vi "Draw Wiggle Trace.vi"(5 "Offsets":cluster{"X offset":u32, "Y offset":u32}, 6 "Trace Options":T1={"Trace Amplitude"=1.0, "Trace Color"=16448250, "Fill options"=enum."No Fill"}, 7 "Plot Area Size":cluster{"Width":u32, "Height":u32}, 8 "error in (no error)":errorcluster, 10 "Data":dbl[][](array[numeric]), 11 "picture in":picture) -> (0 "error out":errorcluster, 3 "picture out":picture)   [LabVIEW 2009]
uses:
  Controls/Trace Options.ctl
  Controls/Fill Options.ctl
  <vilib>/Analysis/baseanly.llb/Quick Scale 2D.vi
  <vilib>/Analysis/NI_AALBase.lvlib
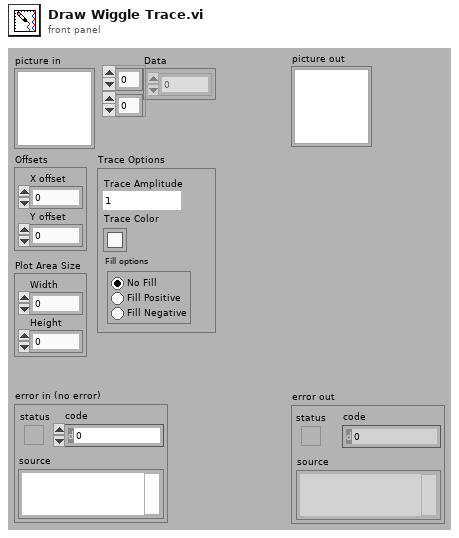
[diagram p1: front panel]
types:
  T1 = typedef "Trace Options.ctl" = cluster{"Trace Amplitude":dbl, "Trace Color":u32, "Fill options":T2}
  T2 = typedef "Fill Options.ctl" = enum32{"No Fill", "Fill Positive", "Fill Negative"}
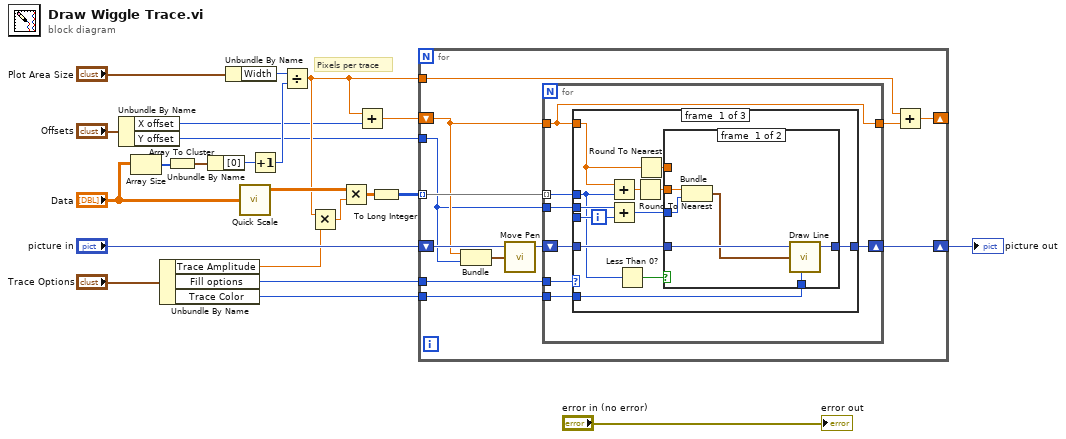
[diagram p0: block diagram]
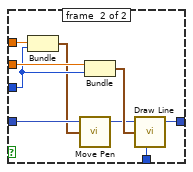
[diagram p2: hidden frame]
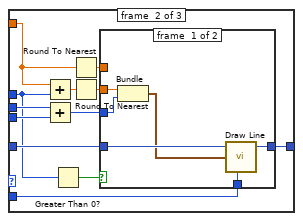
[diagram p3: hidden frame]
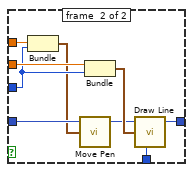
[diagram p4: hidden frame]
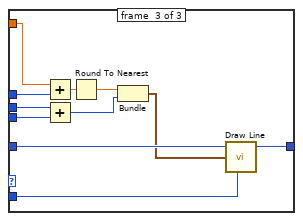
[diagram p5: hidden frame]
diagram:
  # "Pixels per trace"
  n1 = Unbundle By Name("Offsets") -> ("X offset"=w11:u32, "Y offset"=w10:u32)
  n2 = Array Size(array="Data") -> (size(s)=w8:i32[])
  n3 = Unbundle By Name("Trace Options") -> ("Trace Amplitude"=w4:dbl, "Fill options"=w2:T2, "Trace Color"=w1:u32)
  n4 = Array To Cluster(array=w8) -> (cluster=w6:cluster{"[0]":i32, "[1]":i32})
  n5 = Unbundle By Name(w6) -> ("[0]"=w19:i32)
  n6 = Unbundle By Name("Plot Area Size") -> ("Width"=w12:u32)
  n7 = call-poly <vilib>:"Quick Scale.vi"("X"="Data") -> ("Yij=Xij/Max|X|"=w23:dbl[][])  [unwired: 2 out]
  n8 = Increment(x=w19) -> (x+1=w17:i32)
  n9 = Divide(x=w12, y=w17) -> (x/y=w21:dbl)
  n10 = Multiply(x=w21, y=w4) -> (x*y=w22:dbl)
  n11 = Multiply ("Multiply.vi")(x=w23, y=w22) -> (x*y=w15:dbl[][])
  n12 = Add(x=w21, y=w11) -> (x+y=w18:dbl)
  n13 = To Long Integer(number=w15) -> (32bit integer=w14:i32[][])
  n14 = for {
    tunnel: w14 -> [w35] mode=indexing
    tunnel: w21 -> [w32]
    shift-right: [w31] -> _
    shift-left: w18 -> [w28]
    shift-right: [w34] -> w13
    shift-left: "picture in" -> [w30]
    tunnel: w10 -> [w26]
    tunnel: w2 -> [w25]
    tunnel: w1 -> [w24]
    n15 = Bundle(w28, "Y offset"=w26) -> (w27:cluster{dbl, "Y offset":u32})  [unwired: 1 in]
    n16 = call <vilib>:"Move Pen.vi"("new position"=w27, "picture"=w30) -> ("new picture"=w29:picture)  [unwired: 3 in]
    n17 = for {
      tunnel: w35 -> [w39] mode=indexing
      tunnel: w28 -> [w38]
      shift-right: [w43] -> w34
      shift-left: w29 -> [w42]
      tunnel: [w38] -> w33
      tunnel: w26 -> [w40]
      tunnel: w25 -> [w36]
      tunnel: w24 -> [w37]
      i -> [w41]
      n18 = case shown="\"Fill Negative\"" w36 {
        tunnel: [w55 w82 w108] -> w43
        tunnel: w42 -> [w54 w81 w107]
        tunnel: w41 -> [w53 w80 w106]
        tunnel: w40 -> [w51 w78 w104]
        tunnel: w39 -> [w49 w76 w102]
        tunnel: w38 -> [w47 w74 w100]
        tunnel: w37 -> [w45 w72 w99]
        frame #0 {
          n19 = Add(x=w47, y=w49) -> (x+y=w48:dbl)
          n20 = Add(x=w51, y=w53) -> (x+y=w52:u32)
          n21 = Less Than 0?(x=w49) -> (x < 0?=w44:bool)
          n22 = Round To Nearest(number=w48) -> (nearest integer value=w50:dbl)
          n23 = Round To Nearest(number=w47) -> (nearest integer value=w46:dbl)
          n24 = case shown="True" w44 {
            tunnel: [w61 w70] -> w55
            tunnel: w54 -> [w60 w67]
            tunnel: w52 -> [w58 w64]
            tunnel: w50 -> [w57 w68]
            tunnel: w46 -> [_ w65]
            tunnel: w45 -> [w56 w62]
            frame #0 {
              n25 = Bundle(w57, w58) -> (w59:cluster{dbl, u32})  [unwired: 1 in]
              n26 = call <vilib>:"Draw Line.vi"("picture"=w60, "end point"=w59, "color(black)"=w56) -> ("new picture"=w61:picture)  [unwired: 6 in]
            }
            frame #1 {
              n27 = Bundle(w65, w64) -> (w63:cluster{dbl, u32})  [unwired: 1 in]
              n28 = call <vilib>:"Move Pen.vi"("new position"=w63, "picture"=w67) -> ("new picture"=w66:picture)  [unwired: 3 in]
              n29 = Bundle(w68, w64) -> (w69:cluster{dbl, u32})  [unwired: 1 in]
              n30 = call <vilib>:"Draw Line.vi"("picture"=w66, "end point"=w69, "color(black)"=w62) -> ("new picture"=w70:picture)  [unwired: 6 in]
            }
          }
        }
        frame #1 {
          n31 = Add(x=w74, y=w76) -> (x+y=w75:dbl)
          n32 = Add(x=w78, y=w80) -> (x+y=w79:u32)
          n33 = Greater Than 0?(x=w76) -> (x > 0?=w71:bool)
          n34 = Round To Nearest(number=w74) -> (nearest integer value=w73:dbl)
          n35 = Round To Nearest(number=w75) -> (nearest integer value=w77:dbl)
          n36 = case shown="True" w71 {
            tunnel: [w88 w97] -> w82
            tunnel: w81 -> [w87 w94]
            tunnel: w79 -> [w85 w91]
            tunnel: w77 -> [w84 w95]
            tunnel: w73 -> [_ w92]
            tunnel: w72 -> [w83 w89]
            frame #0 {
              n37 = Bundle(w84, w85) -> (w86:cluster{dbl, u32})  [unwired: 1 in]
              n38 = call <vilib>:"Draw Line.vi"("picture"=w87, "end point"=w86, "color(black)"=w83) -> ("new picture"=w88:picture)  [unwired: 6 in]
            }
            frame #1 {
              n39 = Bundle(w92, w91) -> (w90:cluster{dbl, u32})  [unwired: 1 in]
              n40 = call <vilib>:"Move Pen.vi"("new position"=w90, "picture"=w94) -> ("new picture"=w93:picture)  [unwired: 3 in]
              n41 = Bundle(w95, w91) -> (w96:cluster{dbl, u32})  [unwired: 1 in]
              n42 = call <vilib>:"Draw Line.vi"("picture"=w93, "end point"=w96, "color(black)"=w89) -> ("new picture"=w97:picture)  [unwired: 6 in]
            }
          }
        }
        frame #2 {
          n43 = Add(x=w100, y=w102) -> (x+y=w101:dbl)
          n44 = Add(x=w104, y=w106) -> (x+y=w105:u32)
          n45 = Round To Nearest(number=w101) -> (nearest integer value=w103:dbl)
          n46 = Bundle(w103, w105) -> (w98:cluster{dbl, u32})  [unwired: 1 in]
          n47 = call <vilib>:"Draw Line.vi"("picture"=w107, "end point"=w98, "color(black)"=w99) -> ("new picture"=w108:picture)  [unwired: 6 in]
        }
      }
    }
    n48 = Add(x=w32, y=w33) -> (x+y=w31:dbl)
  }
  "picture out" <- w13
  "error out" <- "error in (no error)"
